vi "Initialize Camera.vi"(8 "error in (no error)":errorcluster, 11 "CCDCamera in":refnum<class "Simulated Camera.lvclass">) -> (0 "error out":errorcluster, 3 "CCDCamera out":refnum<class "Simulated Camera.lvclass">)   [LabVIEW 2018, in "Simulated Camera.lvclass"]
doc: "Initialize the camera"
uses:
  Simulated Camera.lvclass
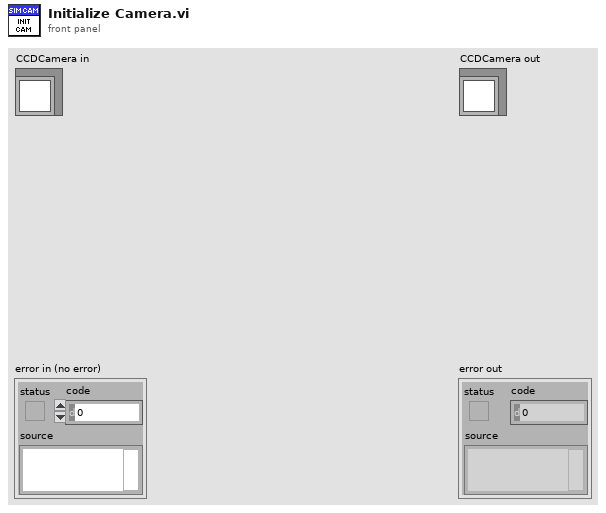
[diagram p1: front panel]
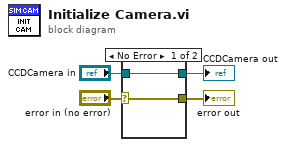
[diagram p0: block diagram]
diagram:
  n1 = case shown="No Error" "error in (no error)" {
    selector: "error in (no error)" -> [w5 w8]
    tunnel: [w5 w8] -> w1
    tunnel: [w6 w7] -> w2
    tunnel: "CCDCamera in" -> [w6 w7]
    frame No Error {
    }
    frame Error {
    }
  }
  "error out" <- w1
  "CCDCamera out" <- w2
